vi "take_and_read_LCD.vi"() -> (0 "Av T":dbl, 2 "Inst. T":dbl, 3 "Image":T2(plugin-control))   [LabVIEW 2017]
uses:
  <vilib>/vision/NI_Vision_Development_Module.lvlib
  <vilib>/Analysis/NI_AALBase.lvlib
panel:
  in  "Image Type":T1 items=["Grayscale (U8)", "Grayscale (I16)", "Grayscale (SGL)", "Complex (CSG)", "RGB (U32)", "HSL (U32)", "RGB (U64)", "Grayscale (U16)"]
  out "Array":dbl[](array[numeric])
  out "Segments status":T3(array[cluster])
  in  "Camera Name":refnum<k21>="cam1" caption="IMAQdx Session"
  in  "File Path":path
  in  "ROI Descriptor out":T4 {"Contours"."Type" items=["No Selection", "Point", "Line", "Rectangle", "Oval", "Polygon", "Free", "Annulus", "Unused2", "Unused3", "Broken Line", "Free Hand Line", "Rotated Rectangle"]}
  in  "stop":bool
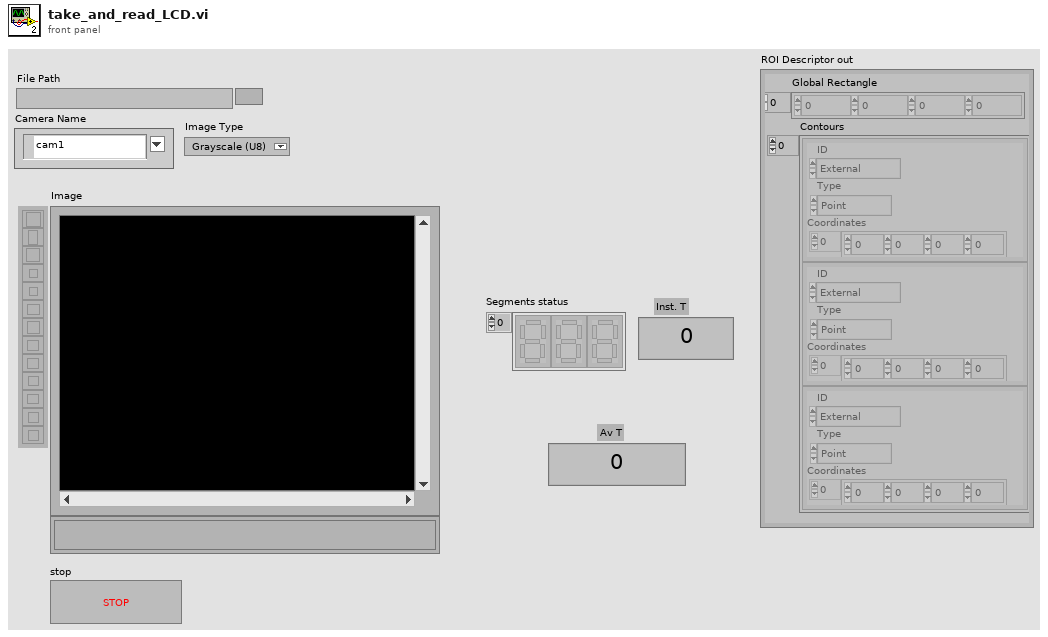
[diagram p1: front panel]
types:
  T1 = typedef "Image Type" = u32
  T2 = typedef "IMAQ Image.ctl" = refnum<image>
  T3 = cluster{bool, bool, bool, bool, bool, bool, bool}[]
  T4 = cluster{"Global Rectangle":i32[], "Contours":cluster{"ID":enum32{"External", "Internal"}, "Type":u32, "Coordinates":i32[]}[]}
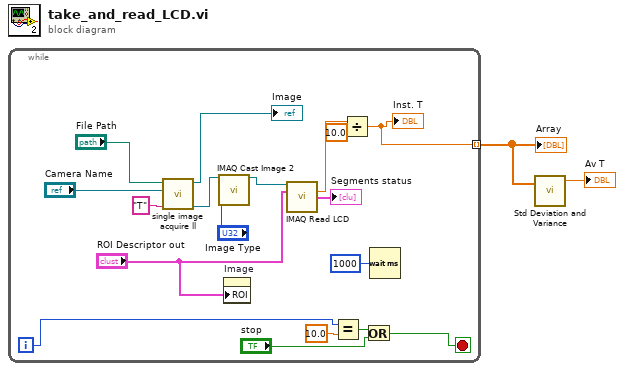
[diagram p0: block diagram]
diagram:
  n1 = while {
    tunnel: [w5] -> w2 mode=indexing
    i -> [w19]
    stop <- w16 stop-if-true
    n2 = call "single image acquire ll.vi"("Image name"="T", "Camera Name"="Camera Name", "File Path"="File Path") -> ("Image Out"=w3:T2, "Image"=→"Image":T2)  [unwired: 7 in]
    n3 = call "IMAQ Cast Image 2"("Image Src"=w3, "Image Type"="Image Type") -> ("Image Dst Out"=w10:T2)  [unwired: 12 in, 1 out]
    n4 = property on="Image" class="ImageControl"("ROI"="ROI Descriptor out") -> ()  [unwired: 2 in, 2 out]
    n5 = call "IMAQ Read LCD"("Image"=w10, "ROI Descriptor"="ROI Descriptor out") -> ("Output value"=w7:dbl, "Segments status"=→"Segments status":T3)  [unwired: 5 in, 7 out]
    n6 = Equal?(x=w19, y=10.0) -> (x = y?=w18:bool)
    n7 = Divide(x=w7, y=10.0) -> (x/y=w5:dbl)
    "Inst. T" <- w5
    n8 = Or(x=w18, y="stop") -> (x .or. y?=w16:bool)
    n9 = Wait (ms)(milliseconds to wait=u32 1000) -> ()  [unwired: 1 out]
  }
  "Array" <- w2
  n10 = call <vilib>:"Std Deviation and Variance.vi"("X"=w2) -> ("mean"=→"Av T":dbl)  [unwired: 1 in, 2 out]
